vi "DriverStationGetData.vi"   [LabVIEW 2019]
doc: "This VI recieves data from the FRC 4265 Dashboard continuously, in all robot modes. These may include safety overrides, calibration commands, and configuration parameters. However this VI should never include standard driver or manipulator commands."
uses:
  f2972b46-d919-4210-bfdf-d3cf9c7f3ddc.vi
  <vilib>/Rock Robotics/Network Tables/NT Read Boolean.vi
  dsdata.vi
  <vilib>/Rock Robotics/Network Tables/NT Read Number.vi
  sensors.vi
  <vilib>/Rock Robotics/Network Tables/NT Read String.vi
  refnums.vi
  GRNF_Joystick.vi
  <vilib>/Utility/xml.llb/Write to XML File(string).vi
types:
  T1 = enum16{"Boot Up", "Camera Override", "Power Port", "Ball Tracking"}
  T2 = typedef "WPI_JoystickDevRef.ctl" = cluster{"Device":T3}
  T3 = typedef "WPI_JoystickDeviceEnum.ctl" = enum16{"USB 0", "USB 1", "USB 2", "USB 3", "USB 4", "USB 5"}
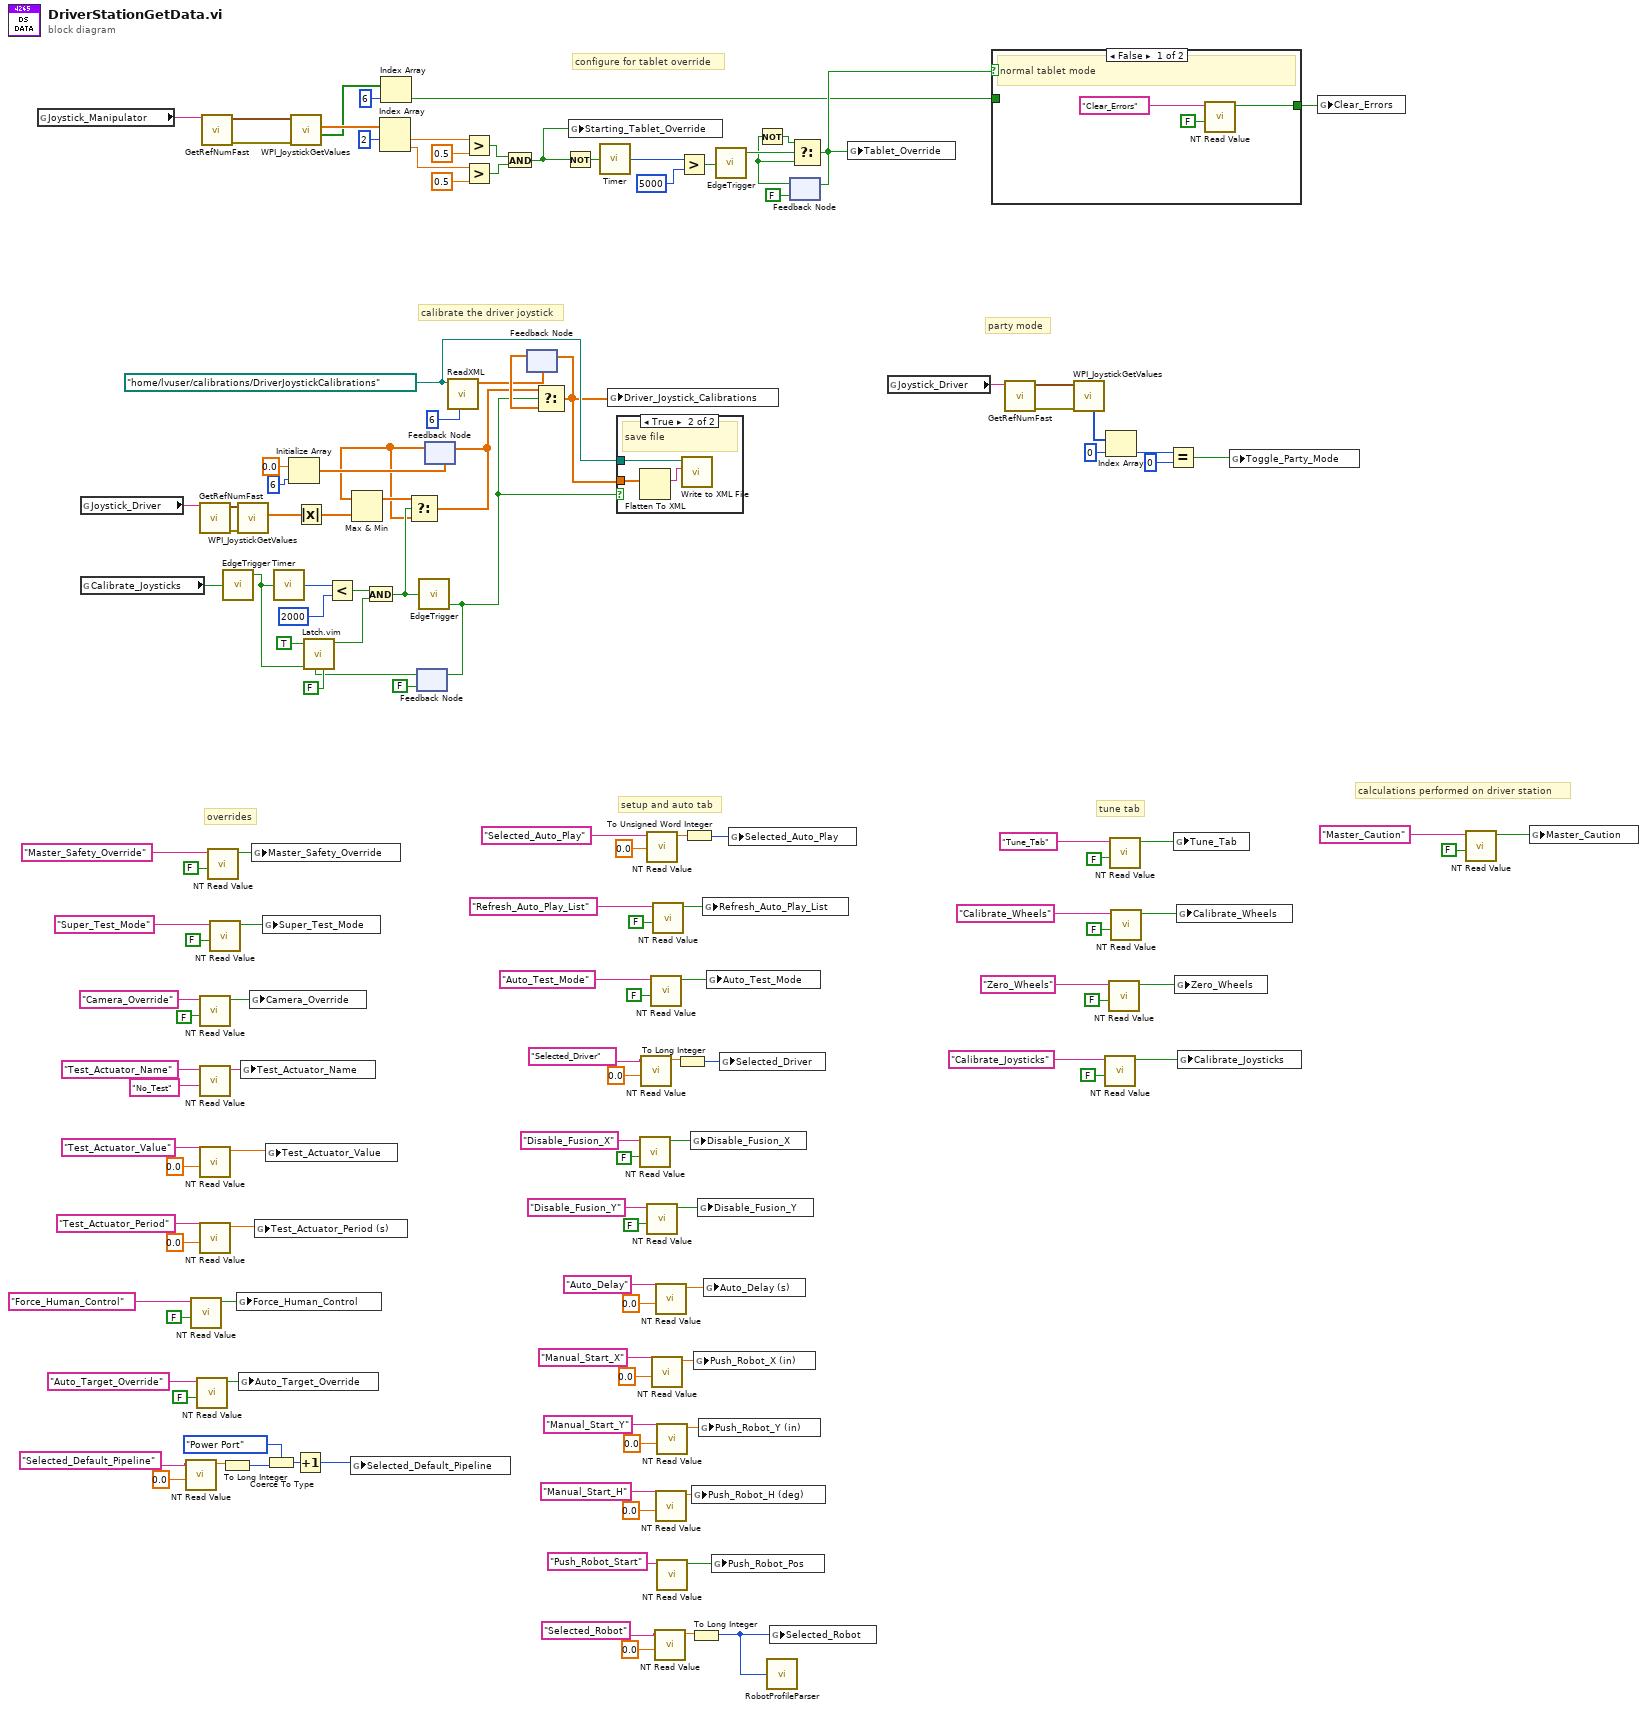
[diagram p0: block diagram]
diagram:
  w56 = path "/home/lvuser/calibrations/DriverJoystickCalibrations" ("path")
  # "party mode"
  # "calibrate the driver joystick"
  # "calculations performed on driver station"
  # "tune tab"
  # "overrides"
  # "setup and auto tab"
  # "configure for tablet override"
  n1 = global read "refnums.vi" "Joystick_Manipulator"() -> (w71:string)
  n2 = global read "refnums.vi" "Joystick_Driver"() -> (w52:string)
  n3 = global read "dsdata.vi" "Calibrate_Joysticks"() -> (w49:bool)
  n4 = call-poly <vilib>:"NT Read Value.vi"("Default Value"=0.0, "Name"="Selected_Default_Pipeline" ("refnum name")) -> ("Numeric"=w14:dbl)  [unwired: 8 in, 1 out]
  n5 = call-poly <vilib>:"NT Read Value.vi"("Default Value"=FALSE, "Name"="Force_Human_Control" ("refnum name")) -> ("Boolean"=w16:bool)  [unwired: 8 in, 1 out]
  n6 = call-poly <vilib>:"NT Read Value.vi"("Default Value"=FALSE, "Name"="Auto_Target_Override" ("refnum name")) -> ("Boolean"=w96:bool)  [unwired: 8 in, 1 out]
  n7 = call-poly "GetRefNumFast.vi"("RefNum Name"=w52) -> ("Error"=w50:errorcluster, "Device Reference"=w51:T2)  [unwired: 5 in]
  n8 = call-poly <vilib>:"NT Read Value.vi"("Default Value"=FALSE, "Name"="Camera_Override" ("refnum name")) -> ("Boolean"=w111:bool)  [unwired: 8 in, 1 out]
  n9 = call-poly <vilib>:"NT Read Value.vi"("Default Value"="No_Test", "Name"="Test_Actuator_Name" ("refnum name")) -> ("String"=w103:string)  [unwired: 8 in, 1 out]
  n10 = call-poly <vilib>:"NT Read Value.vi"("Default Value"=0.0, "Name"="Test_Actuator_Value" ("refnum name")) -> ("Numeric"=w99:dbl)  [unwired: 8 in, 1 out]
  n11 = call-poly <vilib>:"NT Read Value.vi"("Default Value"=0.0, "Name"="Test_Actuator_Period" ("refnum name")) -> ("Numeric"=w24:dbl)  [unwired: 8 in, 1 out]
  n12 = call-poly "GetRefNumFast.vi"("RefNum Name"=w71) -> ("Error"=w72:errorcluster, "Device Reference"=w73:T2)  [unwired: 5 in]
  n13 = call-poly <vilib>:"NT Read Value.vi"("Default Value"=FALSE, "Name"="Master_Safety_Override" ("refnum name")) -> ("Boolean"=w116:bool)  [unwired: 8 in, 1 out]
  n14 = call-poly <vilib>:"NT Read Value.vi"("Default Value"=FALSE, "Name"="Super_Test_Mode" ("refnum name")) -> ("Boolean"=w143:bool)  [unwired: 8 in, 1 out]
  n15 = To Long Integer(number=w14) -> (32bit integer=w11:i32)
  n16 = call "EdgeTrigger.vi"("Input Signal"=w49) -> ("Rising Edge Trigger"=w48:bool)  [unwired: 2 out]
  n17 = global write "dsdata.vi" "Force_Human_Control"(w16) -> ()
  n18 = call <vilib>:"WPI_JoystickGetValues.vi"("error in (no error)"=w50, "JoystickDevRef"=w51) -> ("Axes"=w35:dbl[])  [unwired: 5 in, 4 out]
  n19 = global write "dsdata.vi" "Auto_Target_Override"(w96) -> ()
  n20 = global write "dsdata.vi" "Test_Actuator_Name"(w103) -> ()
  n21 = global write "dsdata.vi" "Camera_Override"(w111) -> ()
  n22 = global write "dsdata.vi" "Master_Safety_Override"(w116) -> ()
  n23 = global write "dsdata.vi" "Test_Actuator_Period (s)"(w24) -> ()
  n24 = global write "dsdata.vi" "Super_Test_Mode"(w143) -> ()
  n25 = global write "dsdata.vi" "Test_Actuator_Value"(w99) -> ()
  n26 = Coerce To Type(0:w11, 1:T1."Power Port" ("Selected_Default_Pipeline")) -> (2:w10:T1)
  n27 = call "Timer.vi"("Reset Timer"=w48) -> ("Time (ms)"=w54:u32)
  n28 = Initialize Array(0.0 ("element"), 6 ("dimension size")) -> (w28:dbl[])
  n29 = call <vilib>:"WPI_JoystickGetValues.vi"("error in (no error)"=w72, "JoystickDevRef"=w73) -> ("Buttons"=w79:bool[], "Axes"=w95:dbl[])  [unwired: 5 in, 3 out]
  n30 = Increment(x=w10) -> (x+1=w9:T1)
  n31 = Absolute Value(x=w35) -> (abs(x)=w32:dbl[])
  n32 = Less?(x=w54, y=u32 2000) -> (x < y?=w45:bool)
  n33 = global write "dsdata.vi" "Selected_Default_Pipeline"(w9) -> ()
  n34 = Index Array(array=w95, index #1=2 ("index")) -> (element #1=w85:dbl, element #2=w84:dbl)  [unwired: 1 in]
  n35 = Index Array(array=w79, index=6) -> (element=w77:bool)
  n36 = feedback #1(FALSE ("Falling Edge Trigger")) -> (w42:bool)
  n37 = call "Latch.vim"("Default Value"=FALSE, "Reset"=w42, "Latch Signal"=w48, "Latch Value"=TRUE) -> ("Latched"=w44:bool)  [unwired: 7 in]
  n38 = And(x=w45, y=w44) -> (x .and. y?=w43:bool)
  n39 = call "EdgeTrigger.vi"("Input Signal"=w43) -> ("Falling Edge Trigger"=w40:bool)  [unwired: 2 out]
  n40 = feedback-in #1(w40) -> ()
  n41 = feedback #2(w28) -> (w27:dbl[])
  n42 = Max & Min(x=w27, y=w32) -> (max(x,y)=w34:dbl[])  [unwired: 1 out]
  n43 = Select(t=w34, s=w43, f=w27) -> (s? t:f=w33:dbl[])
  n44 = feedback-in #2(w33) -> ()
  n45 = call "ReadXML.vi"("Default Number of Elements"=6, "File Path (.xml)"=w56) -> ("Data"=w55:dbl[])  [unwired: 8 in, 1 out]
  n46 = Greater?(x=w85, y=0.5) -> (0:w86:bool)
  n47 = Greater?(x=w84, y=0.5) -> (0:w82:bool)
  n48 = And(x=w86, y=w82) -> (x .and. y?=w60:bool)
  n49 = feedback #3(w55) -> (w57:dbl[])
  n50 = Select(t=w33, s=w40, f=w57) -> (s? t:f=w36:dbl[])
  n51 = feedback-in #3(w36) -> ()
  n52 = Not(x=w60) -> (.not. x?=w59:bool)
  n53 = global write "dsdata.vi" "Starting_Tablet_Override"(w60) -> ()
  n54 = call "Timer.vi"("Reset Timer"=w59) -> ("Time (ms)"=w58:u32)
  n55 = global write "dsdata.vi" "Driver_Joystick_Calibrations"(w36) -> ()
  n56 = case shown="True" w40 {
    tunnel: w56 -> [_ w148]
    tunnel: w36 -> [_ w147]
    frame False {
    }
    frame True {
      # "save file"
      n57 = Flatten To XML(anything=w147) -> (xml string=w146:string)
      n58 = call-poly <vilib>:"Write to XML File.vi"("XML Input"=w146, "XML File Path"=w148) -> ()  [unwired: 7 in, 3 out]
    }
  }
  n59 = call-poly <vilib>:"NT Read Value.vi"("Default Value"=FALSE, "Name"="Disable_Fusion_X" ("refnum name")) -> ("Boolean"=w108:bool)  [unwired: 8 in, 1 out]
  n60 = call-poly <vilib>:"NT Read Value.vi"("Default Value"=0.0, "Name"="Selected_Driver" ("refnum name")) -> ("Numeric"=w132:dbl)  [unwired: 8 in, 1 out]
  n61 = call-poly <vilib>:"NT Read Value.vi"("Default Value"=0.0, "Name"="Selected_Auto_Play" ("refnum name")) -> ("Numeric"=w137:dbl)  [unwired: 8 in, 1 out]
  n62 = call-poly <vilib>:"NT Read Value.vi"("Default Value"=FALSE, "Name"="Disable_Fusion_Y" ("refnum name")) -> ("Boolean"=w105:bool)  [unwired: 8 in, 1 out]
  n63 = call-poly <vilib>:"NT Read Value.vi"("Default Value"=FALSE, "Name"="Auto_Test_Mode" ("refnum name")) -> ("Boolean"=w26:bool)  [unwired: 8 in, 1 out]
  n64 = call-poly <vilib>:"NT Read Value.vi"("Default Value"=0.0, "Name"="Manual_Start_X" ("refnum name")) -> ("Numeric"=w68:dbl)  [unwired: 8 in, 1 out]
  n65 = call-poly <vilib>:"NT Read Value.vi"("Default Value"=FALSE, "Name"="Refresh_Auto_Play_List" ("refnum name")) -> ("Boolean"=w140:bool)  [unwired: 8 in, 1 out]
  n66 = call-poly <vilib>:"NT Read Value.vi"("Default Value"=0.0, "Name"="Selected_Robot" ("refnum name")) -> ("Numeric"=w21:dbl)  [unwired: 8 in, 1 out]
  n67 = call-poly <vilib>:"NT Read Value.vi"("Default Value"=0.0, "Name"="Auto_Delay" ("refnum name")) -> ("Numeric"=w119:dbl)  [unwired: 8 in, 1 out]
  n68 = call-poly <vilib>:"NT Read Value.vi"("Default Value"=0.0, "Name"="Manual_Start_H" ("refnum name")) -> ("Numeric"=w62:dbl)  [unwired: 8 in, 1 out]
  n69 = call-poly <vilib>:"NT Read Value.vi"("Default Value"=0.0, "Name"="Manual_Start_Y" ("refnum name")) -> ("Numeric"=w65:dbl)  [unwired: 8 in, 1 out]
  n70 = call-poly <vilib>:"NT Read Value.vi"("Name"="Push_Robot_Start" ("refnum name")) -> ("Boolean"=w61:bool)  [unwired: 9 in, 1 out]
  n71 = To Long Integer(number=w132) -> (32bit integer=w129:i32)
  n72 = Greater?(x=w58, y=u32 5000) -> (0:w91:bool)
  n73 = To Unsigned Word Integer(number=w137) -> (unsigned 16bit integer=w136:u16)
  n74 = global write "dsdata.vi" "Disable_Fusion_X"(w108) -> ()
  n75 = To Long Integer(number=w21) -> (32bit integer=w19:i32)
  n76 = global write "sensors.vi" "Push_Robot_H (deg)"(w62) -> ()
  n77 = global write "sensors.vi" "Push_Robot_X (in)"(w68) -> ()
  n78 = global write "dsdata.vi" "Disable_Fusion_Y"(w105) -> ()
  n79 = global write "sensors.vi" "Push_Robot_Y (in)"(w65) -> ()
  n80 = global write "dsdata.vi" "Refresh_Auto_Play_List"(w140) -> ()
  n81 = global write "dsdata.vi" "Auto_Delay (s)"(w119) -> ()
  n82 = global write "dsdata.vi" "Auto_Test_Mode"(w26) -> ()
  n83 = global write "sensors.vi" "Push_Robot_Pos"(w61) -> ()
  n84 = call "EdgeTrigger.vi"("Input Signal"=w91) -> ("Rising Edge Trigger"=w90:bool)  [unwired: 2 out]
  n85 = global write "dsdata.vi" "Selected_Driver"(w129) -> ()
  n86 = global write "dsdata.vi" "Selected_Auto_Play"(w136) -> ()
  n87 = call "RobotProfileParser.vi"("Selected Robot"=w19) -> ()
  n88 = global write "dsdata.vi" "Selected_Robot"(w19) -> ()
  n89 = feedback #4(FALSE) -> (w87:bool)
  n90 = Not(x=w87) -> (.not. x?=w89:bool)
  n91 = Select(t=w89, s=w90, f=w87) -> (s? t:f=w80:bool)
  n92 = feedback-in #4(w80) -> ()
  n93 = global write "dsdata.vi" "Tablet_Override"(w80) -> ()
  n94 = global read "refnums.vi" "Joystick_Driver"() -> (w6:string)
  n95 = case shown="False" w80 {
    tunnel: [w149 w152] -> w81
    tunnel: w77 -> [_ w152]
    frame False {
      # "normal tablet mode"
      n96 = call-poly <vilib>:"NT Read Value.vi"("Default Value"=FALSE, "Name"="Clear_Errors" ("refnum name")) -> ("Boolean"=w149:bool)  [unwired: 8 in, 1 out]
    }
    frame True {
      # "manipulator override"
    }
  }
  n97 = call-poly "GetRefNumFast.vi"("RefNum Name"=w6) -> ("Error"=w7:errorcluster, "Device Reference"=w8:T2)  [unwired: 5 in]
  n98 = call <vilib>:"WPI_JoystickGetValues.vi"("error in (no error)"=w7, "JoystickDevRef"=w8) -> ("POVs"=w4:i16[])  [unwired: 5 in, 4 out]
  n99 = call-poly <vilib>:"NT Read Value.vi"("Default Value"=FALSE, "Name"="Calibrate_Joysticks" ("refnum name")) -> ("Boolean"=w37:bool)  [unwired: 8 in, 1 out]
  n100 = Index Array(array=w4, index=0) -> (element=w3:i16)
  n101 = call-poly <vilib>:"NT Read Value.vi"("Default Value"=FALSE, "Name"="Zero_Wheels" ("refnum name")) -> ("Boolean"=w123:bool)  [unwired: 8 in, 1 out]
  n102 = call-poly <vilib>:"NT Read Value.vi"("Default Value"=FALSE, "Name"="Tune_Tab" ("refnum name")) -> ("Boolean"=w130:bool)  [unwired: 8 in, 1 out]
  n103 = call-poly <vilib>:"NT Read Value.vi"("Default Value"=FALSE, "Name"="Calibrate_Wheels" ("refnum name")) -> ("Boolean"=w126:bool)  [unwired: 8 in, 1 out]
  n104 = Equal?(x=w3, y=i16 0) -> (x = y?=w1:bool)
  n105 = global write "dsdata.vi" "Tune_Tab"(w130) -> ()
  n106 = global write "dsdata.vi" "Zero_Wheels"(w123) -> ()
  n107 = global write "dsdata.vi" "Calibrate_Wheels"(w126) -> ()
  n108 = global write "dsdata.vi" "Calibrate_Joysticks"(w37) -> ()
  n109 = global write "dsdata.vi" "Toggle_Party_Mode"(w1) -> ()
  n110 = global write "dsdata.vi" "Clear_Errors"(w81) -> ()
  n111 = call-poly <vilib>:"NT Read Value.vi"("Default Value"=FALSE, "Name"="Master_Caution" ("refnum name")) -> ("Boolean"=w74:bool)  [unwired: 8 in, 1 out]
  n112 = global write "dsdata.vi" "Master_Caution"(w74) -> ()
